vi "Read O3 Flag.vi"(8 "error in":errorcluster, 11 "CRDS Data in":refnum<class "CRDS Data.lvclass">) -> (0 "error out":errorcluster, 2 "O3 Flag":bool, 3 "CRDS Data out":refnum<class "CRDS Data.lvclass">)   [LabVIEW 2011, in "CRDS Data.lvclass"]
uses:
  CRDS Data.lvclass
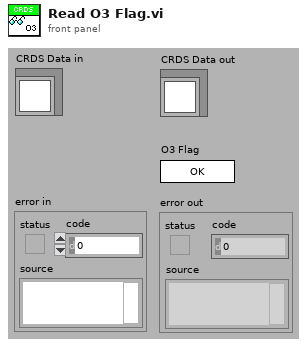
[diagram p1: front panel]
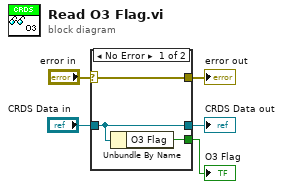
[diagram p0: block diagram]
diagram:
  n1 = case shown="No Error" "error in" {
    selector: "error in" -> [w8 w9]
    tunnel: [w8 w9] -> w4
    tunnel: [w7 w10] -> w2
    tunnel: "CRDS Data in" -> [w7 w10]
    tunnel: [w6 _] -> w1
    frame No Error {
      n2 = Unbundle By Name(w7) -> ("O3 Flag"=w6:bool)
    }
    frame Error {
    }
  }
  "error out" <- w4
  "CRDS Data out" <- w2
  "O3 Flag" <- w1
